vi "Server_L.vi"(8 "stop":bool, 9 "port":u16=13078, 10 "Wait(ms)":i32=500, 11 "Server Name":string="TCPService") -> ()   [LabVIEW 2011]
panel:
  out "error out":errorcluster
  in  "error in":errorcluster
  out "Host_IP":string
  out "Users":i32 caption="#Users"
  out "Active":bool
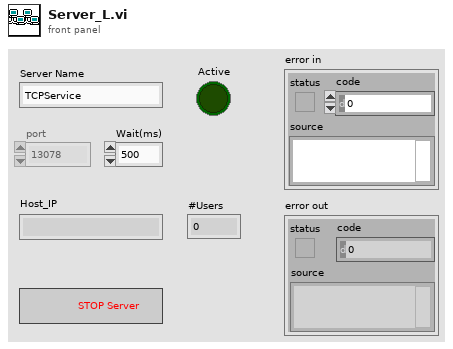
[diagram p1: front panel]
types:
  T1 = cluster{"rem addr":string, "conn ID":refnum<k5>}[]
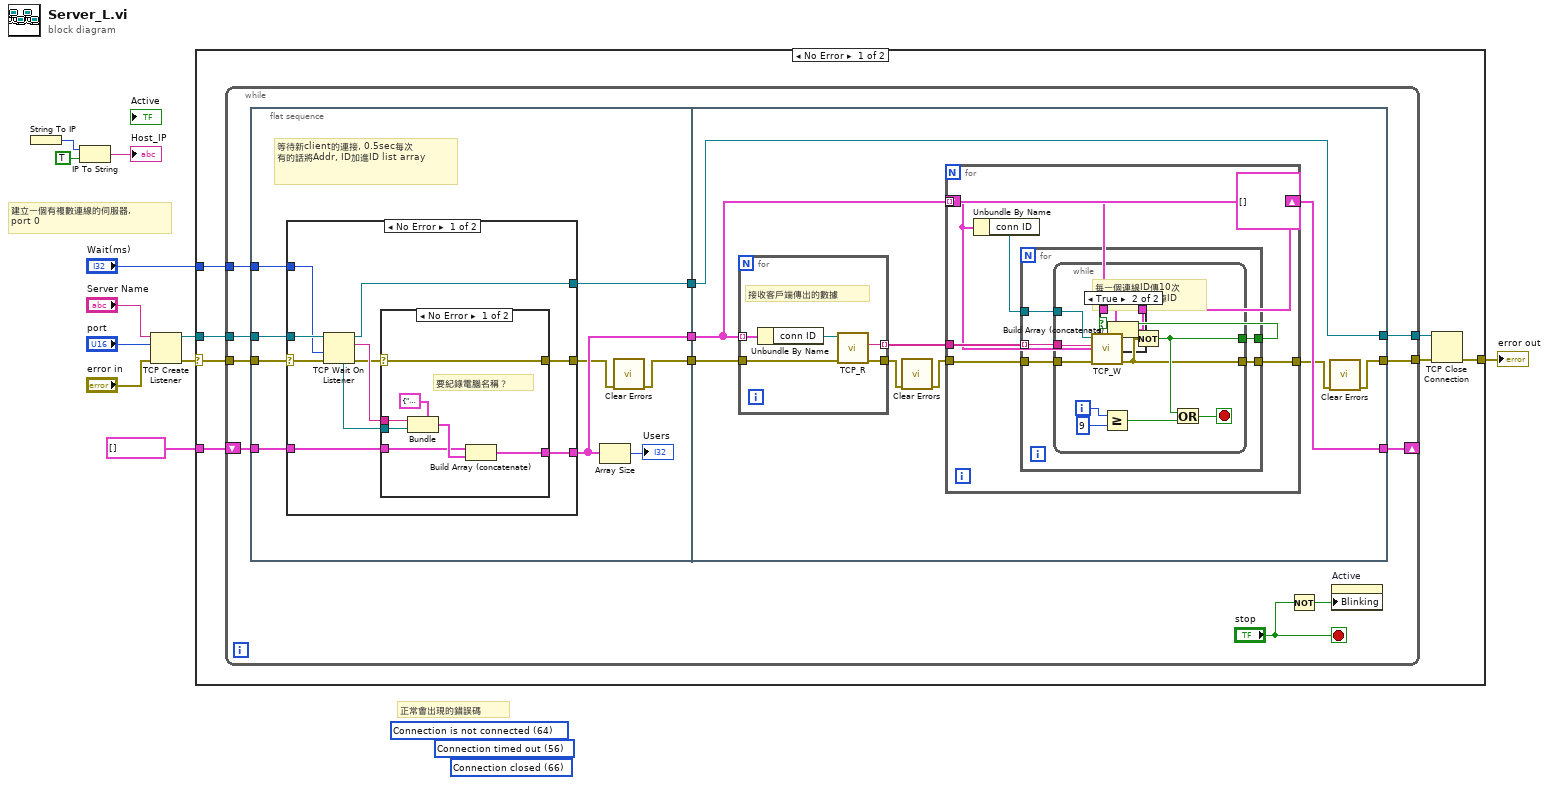
[diagram p0: block diagram]
diagram:
  (unwired) 56 items=["No Error", "Argument Error", "Memory Full", "Out of Zone", "End of File", "File Already Open", "Generic File IO Error", "File Not Found", "File Permission Error", "Disk Full", "Duplicate Path", "Too Many Files Open", "Not Enabled", "Resource File Not Found", "Cannot Add Resource", "Resource Not Found", "Image Not Found", "Image Memory Error", "Pen Does Not Exist", "Config Bad Type", "Config Token Not Found", "Config Parse Error", "Config Memory Error", "Bad External Code Format", "Bad External Code Offset", "External Code Not Present", "Null Window", "Destroy Window Mixup", "Null Menu", "Print Aborted", "Bad Print Record", "Print Driver Error", "Windows Error During Print", "Memory Error During Print", "Print Dialog Error", "Generic Print Error", "Invalid Device Refnum", "Device Not Found", "Device Parameter Error", "Device Unit Error", "Can't Open Device", "Device Call Aborted", "Generic Error", "Cancelled By User", "Object ID Too Low", "Object ID Too High", "Object Not In Heap", "Unknown Heap", "Bad DefProc ID", "DefProc Not In Table", "Message Out Of Range", "Null Method", "Unknown Message", "Manager Call Not Supported", "Bad address", "Connection In progress", "Connection timed out", "Connection is already in progress", "Network attribute not supported", "Network error", "Address in use", "System out of memory", "Connection aborted", "Connection refused", "Connection is not connected", "Connection is already connected", "Connection closed", "Initialize error (interapplication manager)", "Bad occurrence", "Wait on unbound occurrence handler", "Occurrence queue overflow", "Bad path", "Semaphore not signaled", "Unrecognized type (interapplication manager)"] ("2nd Error to Convert")
  (unwired) 66 items=["No Error", "Argument Error", "Memory Full", "Out of Zone", "End of File", "File Already Open", "Generic File IO Error", "File Not Found", "File Permission Error", "Disk Full", "Duplicate Path", "Too Many Files Open", "Not Enabled", "Resource File Not Found", "Cannot Add Resource", "Resource Not Found", "Image Not Found", "Image Memory Error", "Pen Does Not Exist", "Config Bad Type", "Config Token Not Found", "Config Parse Error", "Config Memory Error", "Bad External Code Format", "Bad External Code Offset", "External Code Not Present", "Null Window", "Destroy Window Mixup", "Null Menu", "Print Aborted", "Bad Print Record", "Print Driver Error", "Windows Error During Print", "Memory Error During Print", "Print Dialog Error", "Generic Print Error", "Invalid Device Refnum", "Device Not Found", "Device Parameter Error", "Device Unit Error", "Can't Open Device", "Device Call Aborted", "Generic Error", "Cancelled By User", "Object ID Too Low", "Object ID Too High", "Object Not In Heap", "Unknown Heap", "Bad DefProc ID", "DefProc Not In Table", "Message Out Of Range", "Null Method", "Unknown Message", "Manager Call Not Supported", "Bad address", "Connection In progress", "Connection timed out", "Connection is already in progress", "Network attribute not supported", "Network error", "Address in use", "System out of memory", "Connection aborted", "Connection refused", "Connection is not connected", "Connection is already connected", "Connection closed", "Initialize error (interapplication manager)", "Bad occurrence", "Wait on unbound occurrence handler", "Occurrence queue overflow", "Bad path", "Semaphore not signaled", "Unrecognized type (interapplication manager)"] ("3rd Error to Convert")
  (unwired) 64 items=["No Error", "Argument Error", "Memory Full", "Out of Zone", "End of File", "File Already Open", "Generic File IO Error", "File Not Found", "File Permission Error", "Disk Full", "Duplicate Path", "Too Many Files Open", "Not Enabled", "Resource File Not Found", "Cannot Add Resource", "Resource Not Found", "Image Not Found", "Image Memory Error", "Pen Does Not Exist", "Config Bad Type", "Config Token Not Found", "Config Parse Error", "Config Memory Error", "Bad External Code Format", "Bad External Code Offset", "External Code Not Present", "Null Window", "Destroy Window Mixup", "Null Menu", "Print Aborted", "Bad Print Record", "Print Driver Error", "Windows Error During Print", "Memory Error During Print", "Print Dialog Error", "Generic Print Error", "Invalid Device Refnum", "Device Not Found", "Device Parameter Error", "Device Unit Error", "Can't Open Device", "Device Call Aborted", "Generic Error", "Cancelled By User", "Object ID Too Low", "Object ID Too High", "Object Not In Heap", "Unknown Heap", "Bad DefProc ID", "DefProc Not In Table", "Message Out Of Range", "Null Method", "Unknown Message", "Manager Call Not Supported", "Bad address", "Connection In progress", "Connection timed out", "Connection is already in progress", "Network attribute not supported", "Network error", "Address in use", "System out of memory", "Connection aborted", "Connection refused", "Connection is not connected", "Connection is already connected", "Connection closed", "Initialize error (interapplication manager)", "Bad occurrence", "Wait on unbound occurrence handler", "Occurrence queue overflow", "Bad path", "Semaphore not signaled", "Unrecognized type (interapplication manager)"] ("1st Error to Convert")
  # "正常會出現的錯誤碼"
  # "建立一個有複數連線的伺服器,\nport 0"
  n1 = String To IP() -> (0:w8:u32)  [unwired: 1 in]
  n2 = IP To String(1:TRUE ("dot notation? (F)"), 2:w8) -> (0:→"Host_IP":string)
  n3 = TCP Create Listener(8:"error in", 10:"port", 11:"Server Name") -> (0:w10:errorcluster, 3:w9:refnum<k5>)  [unwired: 2 in, 1 out]
  n4 = case shown="No Error" w10 {
    selector: w10 -> [w16 w102]
    tunnel: w9 -> [w18 _]
    tunnel: T1 [] ("array") -> [w17 _]
    tunnel: [w12 w102] -> w2
    tunnel: "Wait(ms)" -> [w13 _]
    frame No Error {
      n5 = while {
        shift-right: [w27] -> _
        shift-left: w17 -> [w29]
        tunnel: w16 -> [w30]
        tunnel: w18 -> [w28]
        tunnel: [w24] -> w14
        tunnel: [w23] -> w15
        tunnel: w13 -> [w19]
        stop <- "stop" stop-if-true
        n6 = flat-sequence {
          tunnel: w30 -> [w38]
          tunnel: w29 -> [w39]
          tunnel: w28 -> [w37]
          tunnel: [w32] -> w22
          tunnel: [w35] -> w21
          tunnel: [w33] -> w20
          tunnel: w19 -> [w31]
          tunnel: [w69] -> w27
          tunnel: [w63] -> w24
          tunnel: [w62] -> w23
          tunnel: w22 -> [w62]
          tunnel: w21 -> [w68]
          tunnel: w20 -> [w64]
          frame #0 {
            # "等待新client的連接, 0.5sec每次\n有的話將Addr, ID加進ID list array"
            n7 = case shown="No Error" w38 {
              selector: w38 -> [w48 w60]
              tunnel: w37 -> [w49 _]
              tunnel: [w41 w60] -> w34
              tunnel: [w47 _] -> w32
              tunnel: [w46 w59] -> w35
              tunnel: w39 -> [w45 w59]
              tunnel: w31 -> [w40 _]
              frame No Error {
                n8 = TCP Wait On Listener(8:w48, 9:w40, 11:w49) -> (0:w42:errorcluster, 2:w43:string, 3:w47:refnum<k5>, 4:w44:refnum<k5>)  [unwired: 1 in, 1 out]
                n9 = case shown="No Error" w42 {
                  selector: w42 -> [w50 w57]
                  tunnel: [w56 w58] -> w46
                  tunnel: w45 -> [w54 w58]
                  tunnel: w44 -> [w51 _]
                  tunnel: w43 -> [w53 _]
                  tunnel: [w50 w57] -> w41
                  frame No Error {
                    # "要紀錄電腦名稱？"
                    n10 = Bundle(cluster=cluster{"rem addr":string, "conn ID":refnum<k5>} {"rem addr"="", "conn ID"=refnum}, "rem addr"=w53, "conn ID"=w51) -> (w55:cluster{"rem addr":string, "conn ID":refnum<k5>})
                    n11 = Build Array (concatenate)(w54, w55) -> (w56:T1)
                  }
                  frame Error {
                  }
                }
              }
              frame Error {
              }
            }
            n12 = Array Size(array=w35) -> (size(s)=→"Users":i32)
            n13 = call <vilib>:"Clear Errors.vi"("error in (no error)"=w34) -> ("error out"=w33:errorcluster)  [unwired: 5 in, 1 out]
          }
          frame #1 {
            n14 = for {
              tunnel: w68 -> [w101] mode=indexing
              tunnel: [w98] -> w70 mode=indexing
              tunnel: [w99] -> w67
              tunnel: w64 -> [w97]
              # "接收客戶端傳出的數據"
              n15 = Unbundle By Name(w101) -> ("conn ID"=w100:refnum<k5>)
              n16 = call "TCP_R.vi"("error in"=w97, "connection ID"=w100) -> ("error out"=w99:errorcluster, "data out"=w98:string)  [unwired: 7 in, 1 out]
            }
            n17 = call <vilib>:"Clear Errors.vi"("error in (no error)"=w67) -> ("error out"=w66:errorcluster)  [unwired: 5 in, 1 out]
            n18 = for {
              tunnel: w70 -> [w77]
              tunnel: w68 -> [w76] mode=indexing
              tunnel: w66 -> [w74]
              tunnel: [w73] -> w65
              shift-right: [w71] -> w69
              shift-left: T1 [] ("Array") -> [w72]
              n19 = Unbundle By Name(w76) -> ("conn ID"=w78:refnum<k5>)
              n20 = for {
                tunnel: w78 -> [w87]
                tunnel: w77 -> [w86] mode=indexing
                tunnel: [w85] -> w75
                tunnel: w74 -> [w84]
                tunnel: [w83] -> w73
                n21 = while {
                  tunnel: w87 -> [w92]
                  tunnel: w86 -> [w93]
                  tunnel: [w94] -> w85
                  tunnel: w84 -> [w91]
                  tunnel: [w90] -> w83
                  i -> [w89]
                  stop <- w96 stop-if-true
                  # "每一個連線ID傳10次\n都傳不出去就砍掉ID"
                  n22 = call "TCP_W.vi"("error in"=w91, "data in"=w93, "connection ID"=w92) -> ("error IO"=w90:errorcluster)  [unwired: 7 in, 1 out]
                  n23 = Greater Or Equal?(x=w89, y=9 ("x")) -> (x >= y?=w95:bool)
                  n24 = Not(x=w90) -> (.not. x?=w94:bool)
                  n25 = Or(x=w94, y=w95) -> (x .or. y?=w96:bool)
                }
              }
              n26 = case shown="True" w75 {
                tunnel: w72 -> [w79 w81]
                tunnel: w76 -> [_ w80]
                tunnel: [w79 w82] -> w71
                frame False {
                }
                frame True {
                  n27 = Build Array (concatenate)(w81, w80) -> (w82:T1)
                }
              }
            }
            n28 = call <vilib>:"Clear Errors.vi"("error in (no error)"=w65) -> ("error out"=w63:errorcluster)  [unwired: 5 in, 1 out]
          }
        }
        n29 = Not(x="stop") -> (.not. x?=w26:bool)
        n30 = property on="Active" class="Bool (strict)"("Blinking"=w26) -> ()  [unwired: 2 in, 2 out]
      }
      n31 = TCP Close Connection(connection ID=w15, error in (no error)=w14) -> (error out=w12:errorcluster)  [unwired: 1 in, 1 out]
    }
    frame Error {
    }
  }
  "error out" <- w2
